vi "FXPtoSGL_EncodeU32.vi"(0 "FXP 64.24":fxp<+/-,64,24> format="%#_11f") -> (5 "SGL as U32":u32)   [LabVIEW 2011]
uses:
  <vilib>/Platform/TimedLoop/XDataNode/timing_clust.ctl
  <vilib>/Platform/TimedLoop/XDataNode/nitl_modes.ctl
  <vilib>/Platform/TimedLoop/XDataNode/wakeup.ctl
  <vilib>/Platform/TimedLoop/XDataNode/XDataNode.xnode
  <vilib>/Platform/TimedLoop/XDataNode/XDNodeRunTimeDep.lvlib
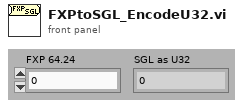
[diagram p1: front panel]
types:
  T1 = typedef "XDNodeRunTimeDep.lvlib/timing_clust.ctl" = cluster{"Expected End [f-1]":u64, "Actual End [f-1]":u64, "Finished Late? [f-1]":bool, "Expected End [i-1]":u64, "Actual End [i-1]":u64, "Finished Late? [i-1]":bool, "Expected Start [i]":u64, "Actual Start [i]":u64, "Expected Start [f]":u64, "Actual Start [f]":u64, "Source Name":string, "Structure Name":string, "Period":i64, "Deadline":i64, "Offset":i64, "Start":i64, "Priority":i32, "Timeout":i32, "Mode":T2, "Wakeup Reason":T3, "Error":errorcluster, "Source Type":string, "Secondary Source Type":string, "Global End Time":u64, "Global Start Time":u64, "Frame Duration":u64, "Iteration Duration":u64, "Assigned CPU":i32, "I/O Scan Engine Mode":u32}
  T2 = typedef "XDNodeRunTimeDep.lvlib/nitl_modes.ctl" = enum32{"No Change", "Process missed periods, maintain original phase", "Discard missed periods, maintain original phase", "Process missed periods, ignore original phase", "Discard missed periods, ignore original phase"}
  T3 = typedef "XDNodeRunTimeDep.lvlib/wakeup.ctl" = enum32{"Normal", "Aborted", "Asynchronous wakeup", "Timing source error", "Timed loop error", "Timeout"}
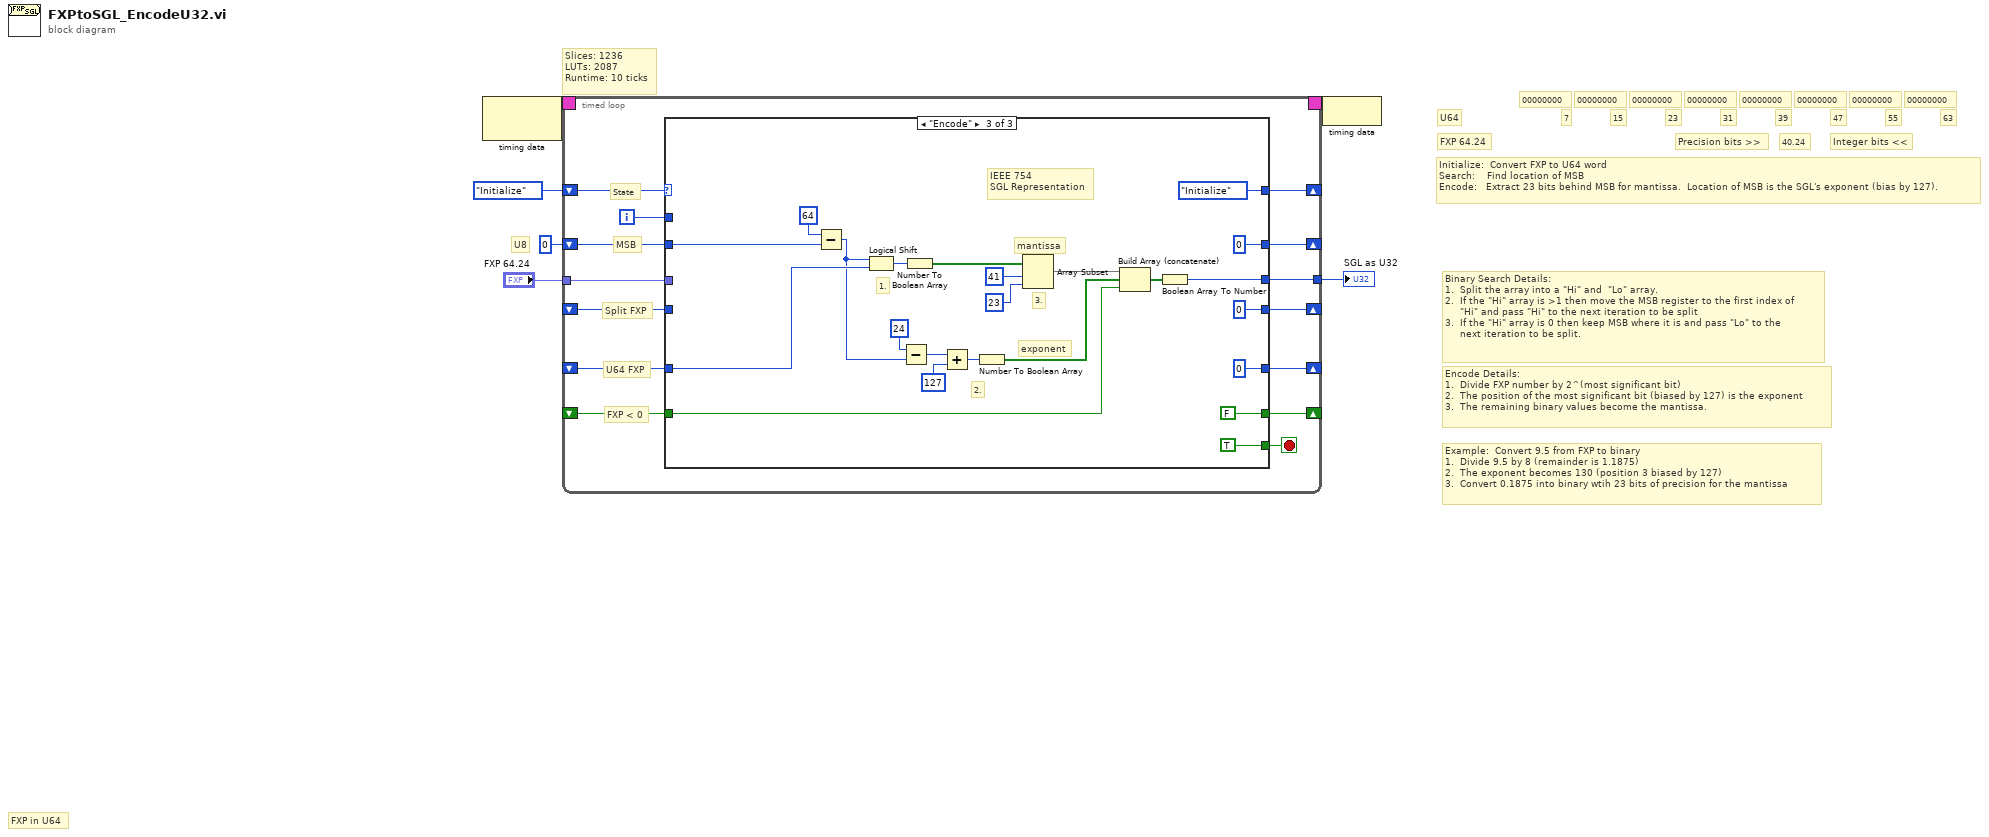
[diagram p0: block diagram]
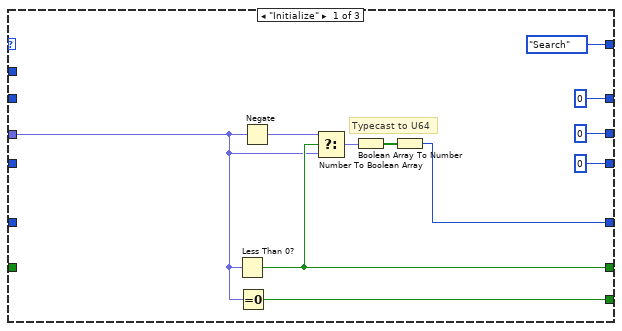
[diagram p2: hidden frame]
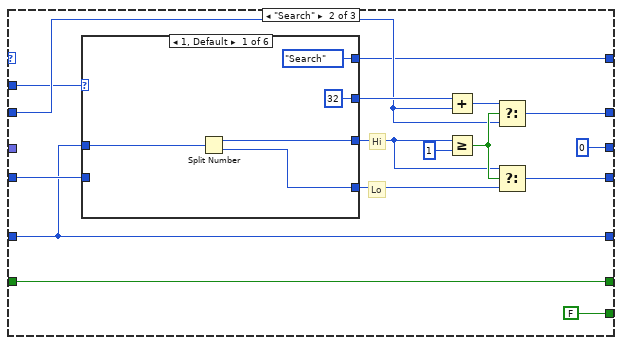
[diagram p3: hidden frame]
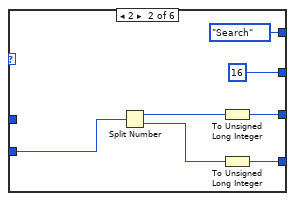
[diagram p4: hidden frame]
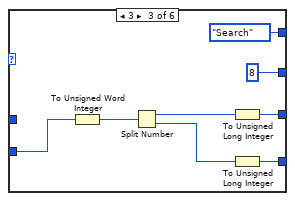
[diagram p5: hidden frame]
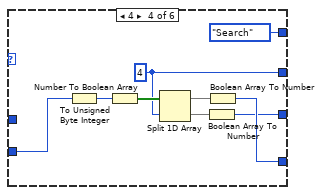
[diagram p6: hidden frame]
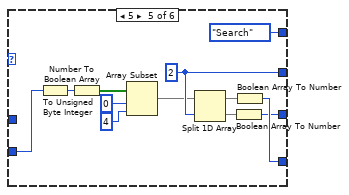
[diagram p7: hidden frame]
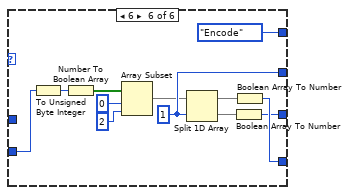
[diagram p8: hidden frame]
diagram:
  # "Binary Search Details:\n1.  Split the array into a \"Hi\" and  \"Lo\" array.\n2.  If the \"Hi\" array is >1 then move the MSB register to the first index of \n     \"Hi\" and pass \"Hi\" to the next iteration to be split\n3.  If the \"Hi\" array is 0 then keep MSB where it is and pass \"Lo\" to the \n     next iteration to be split."
  # "Integer bits <<"
  # "Precision bits >>"
  # "FXP 64.24"
  # "U64"
  # "40.24"
  # "Initialize:  Convert FXP to U64 word\nSearch:    Find location of MSB\nEncode:   Extract 23 bits behind MSB for mantissa.  Location of MSB is the SGL's exponent (bias by 127)."
  # "63"
  # "55"
  # "47"
  # "39"
  # "31"
  # "23"
  # "15"
  # "7"
  # "00000000"
  # "00000000"
  # "00000000"
  # "00000000"
  # "00000000"
  # "00000000"
  # "00000000"
  # "00000000"
  # "U8"
  # "FXP in U64"
  # "Slices: 1236\nLUTs: 2087\nRuntime: 10 ticks"
  # "Example:  Convert 9.5 from FXP to binary\n1.  Divide 9.5 by 8 (remainder is 1.1875) \n2.  The exponent becomes 130 (position 3 biased by 127)\n3.  Convert 0.1875 into binary wtih 23 bits of precision for the mantissa"
  # "Encode Details:\n1.  Divide FXP number by 2^(most significant bit)\n2.  The position of the most significant bit (biased by 127) is the exponent\n3.  The remaining binary values become the mantissa."
  n1 = node-c288() -> (w6:T1)  [unwired: 1 out]
  n2 = timed-loop {
    shift-right: [w20] -> _
    shift-left: u8 0 -> [w16]
    timing: w6 -> [_]
    timing-out: [_] -> w5
    tunnel: "FXP 64.24" -> [w19]
    shift-right: [w18] -> _
    shift-left: _ -> [w17]
    shift-right: [w14] -> _
    shift-left: enum16{"Initialize", "Search", "Encode"}."Initialize" ("Enum") -> [w15]
    tunnel: [w12] -> w1
    shift-right: [w11] -> _
    shift-left: _ -> [w10]
    shift-right: [w9] -> _
    shift-left: _ -> [w8]
    i -> [w7]
    stop <- w13 stop-if-true
    # "Split FXP"
    # "U64 FXP"
    # "MSB"
    # "FXP < 0"
    # "State"
    n3 = case shown="\"Encode\"" w15 {
      tunnel: w16 -> [_ w40 w102]
      tunnel: [u8 0 ("Low") w39 u8 0 ("Low")] -> w20
      tunnel: w19 -> [w29 _ _]
      tunnel: [w30 w45 FALSE] -> w18
      tunnel: w17 -> [_ w45 w115]
      tunnel: [enum16{"Initialize", "Search", "Encode"}."Search" ("Enum") w36 enum16{"Initialize", "Search", "Encode"}."Initialize" ("Enum")] -> w14
      tunnel: [w22 FALSE TRUE] -> w13
      tunnel: [u32 0 ("f") u32 0 ("f") w101] -> w12
      tunnel: [w24 w34 u64 0] -> w11
      tunnel: w10 -> [_ w34 w106]
      tunnel: [u32 0 w38 u32 0] -> w9
      tunnel: w8 -> [_ w37 _]
      tunnel: w7 -> [_ w35 _]
      frame "Initialize" {
        # "Typecast to U64"
        n4 = Less Than 0?(x=w29) -> (x < 0?=w30:bool)
        n5 = Equal To 0?(x=w29) -> (x = 0?=w22:bool)
        n6 = Negate(x=w29) -> (-x=w25:fxp<+/-,64,24>)
        n7 = Select(t=w25, s=w30, f=w29) -> (s? t:f=w26:fxp<+/-,64,24>)
        n8 = Number To Boolean Array(number=w26) -> (Boolean array=w21:bool[])
        n9 = Boolean Array To Number(Boolean array=w21) -> (number=w24:u64)
      }
      frame "Search" {
        # "Lo"
        # "Hi"
        n10 = case shown="1, Default" w35 {
          tunnel: [w49 w56 w64 w73 w86 w98] -> w33
          tunnel: [w48 w54 w63 w72 w85 w97] -> w32
          tunnel: w37 -> [_ w57 w67 w69 w84 w96]
          tunnel: [u8 32 ("index") u8 16 ("index") u8 8 ("index") w71 w82 w94] -> w41
          tunnel: [enum16{"Initialize", "Search", "Encode"}."Search" ("Enum") enum16{"Initialize", "Search", "Encode"}."Search" ("Enum") enum16{"Initialize", "Search", "Encode"}."Search" ("Enum") enum16{"Initialize", "Search", "Encode"}."Search" ("Enum") enum16{"Initialize", "Search", "Encode"}."Search" ("Enum") enum16{"Initialize", "Search", "Encode"}."Encode" ("Enum")] -> w36
          tunnel: w34 -> [w50 _ _ _ _ _]
          frame 1, Default {
            n11 = Split Number(x=w50) -> (hi(x)=w48:u32, lo(x)=w49:u32)
          }
          frame 2 {
            n12 = Split Number(x=w57) -> (hi(x)=w53:u16, lo(x)=w55:u16)
            n13 = To Unsigned Long Integer(number=w53) -> (unsigned 32bit integer=w54:u32)
            n14 = To Unsigned Long Integer(number=w55) -> (unsigned 32bit integer=w56:u32)
          }
          frame 3 {
            n15 = To Unsigned Word Integer(number=w67) -> (unsigned 16bit integer=w61:u16)
            n16 = Split Number(x=w61) -> (hi(x)=w60:u8, lo(x)=w62:u8)
            n17 = To Unsigned Long Integer(number=w60) -> (unsigned 32bit integer=w63:u32)
            n18 = To Unsigned Long Integer(number=w62) -> (unsigned 32bit integer=w64:u32)
          }
          frame 4 {
            w71 = u8 4 ("index")
            n19 = To Unsigned Byte Integer(number=w69) -> (unsigned 8bit integer=w68:u8)
            n20 = Number To Boolean Array(number=w68) -> (Boolean array=w76:bool[])
            n21 = Split 1D Array(array=w76, index=w71) -> (first subarray=w75:bool[], second subarray=w74:bool[])
            n22 = Boolean Array To Number(Boolean array=w74) -> (number=w72:u32)
            n23 = Boolean Array To Number(Boolean array=w75) -> (number=w73:u32)
          }
          frame 5 {
            w82 = u8 2 ("index")
            n24 = To Unsigned Byte Integer(number=w84) -> (unsigned 8bit integer=w83:u8)
            n25 = Number To Boolean Array(number=w83) -> (Boolean array=w79:bool[])
            n26 = Array Subset(array=w79, index=0, length=4) -> (w78:bool[])
            n27 = Split 1D Array(array=w78, index=w82) -> (first subarray=w88:bool[], second subarray=w87:bool[])
            n28 = Boolean Array To Number(Boolean array=w87) -> (number=w85:u32)
            n29 = Boolean Array To Number(Boolean array=w88) -> (number=w86:u32)
          }
          frame 6 {
            w94 = u8 1 ("index")
            n30 = To Unsigned Byte Integer(number=w96) -> (unsigned 8bit integer=w95:u8)
            n31 = Number To Boolean Array(number=w95) -> (Boolean array=w91:bool[])
            n32 = Array Subset(array=w91, index=0, length=2) -> (w90:bool[])
            n33 = Split 1D Array(array=w90, index=w94) -> (first subarray=w100:bool[], second subarray=w99:bool[])
            n34 = Boolean Array To Number(Boolean array=w99) -> (number=w97:u32)
            n35 = Boolean Array To Number(Boolean array=w100) -> (number=w98:u32)
          }
        }
        n36 = Add(x=w41, y=w40) -> (x+y=w44:u8)
        n37 = Greater Or Equal?(x=w32, y=u32 1) -> (x >= y?=w43:bool)
        n38 = Select(t=w44, s=w43, f=w40) -> (s? t:f=w39:u8)
        n39 = Select(t=w32, s=w43, f=w33) -> (s? t:f=w38:u32)
      }
      frame "Encode" {
        # "3."
        # "2."
        # "1."
        # "IEEE 754\nSGL Representation"
        # "mantissa"
        # "exponent"
        n40 = Subtract(x=u8 64 ("y"), y=w102) -> (x-y=w103:u8)
        n41 = Logical Shift(y=w103, x=w106) -> (x << y=w109:u64)
        n42 = Subtract(x=u8 24 ("y"), y=w103) -> (x-y=w111:u8)
        n43 = Number To Boolean Array(number=w109) -> (Boolean array=w117:bool[])
        n44 = Add(x=w111, y=u8 127) -> (x+y=w122:u8)
        n45 = Number To Boolean Array(number=w122) -> (Boolean array=w121:bool[])
        n46 = Array Subset(array=w117, index=41, length=23 ("y")) -> (w108:bool[])
        n47 = Build Array (concatenate)(w108, w121, w115) -> (w120:bool[])
        n48 = Boolean Array To Number(Boolean array=w120) -> (number=w101:u32)
      }
    }
  }
  "SGL as U32" <- w1
  n49 = node-c288(w5) -> ()
